vi "Prompt for Step.vi"(8 "error in (no error)":errorcluster, 10 "Subpanel Ref":refnum<vi>, 11 "Numeric Assertion in":refnum<class "Numeric Assertion.lvclass">) -> (0 "error out":errorcluster, 3 "Numeric Assertion out":refnum<class "Numeric Assertion.lvclass">)   [LabVIEW 2020, in "MacroAssert.lvlib" / "Numeric Assertion.lvclass"]
doc: "Displays its own window into <B>Subpanel Ref</B> for the user to enter a macro step."
uses:
  Numeric Assertion.lvclass
  Assertion Step/Assertion Step.lvclass
panel:
  out "Subtype Description":string
  in  "Comparison Value":dbl
  in  "Comparison Type":u16(ring) items=["Equals", "Is greater than", "Is greater than or equal to", "Is less than", "Is less than or equal to", "Does not equal"]
  in  "Step Subtype":u16(ring) items=["Numeric Ctl Value", "Array Ctl Size", "Ctl Width Property", "Ctl Height Property", "VI Width", "VI Height", "Window Width", "Window Height", "Window Scale"]
  in  "Object Name":string
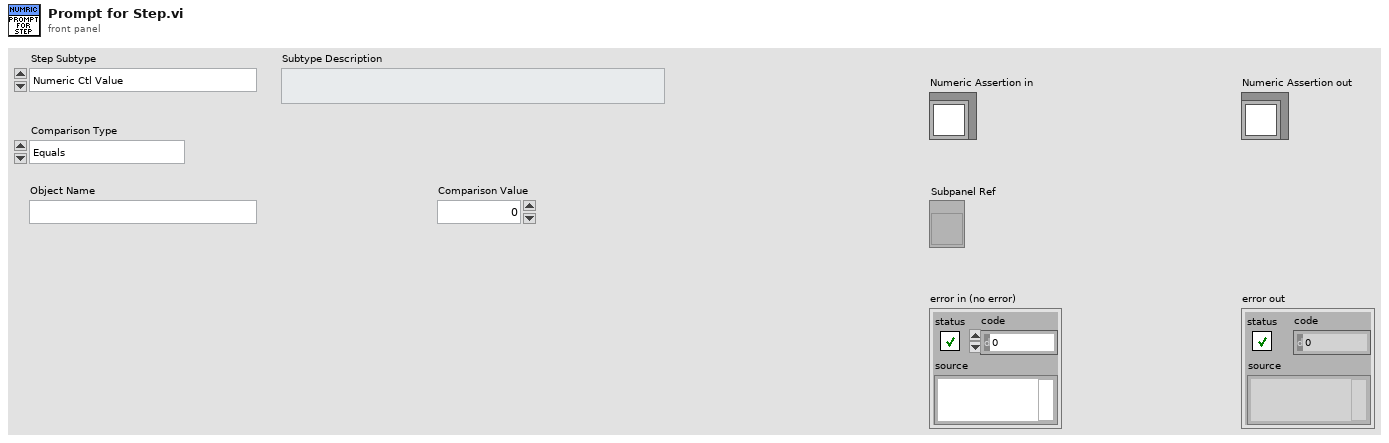
[diagram p1: front panel]
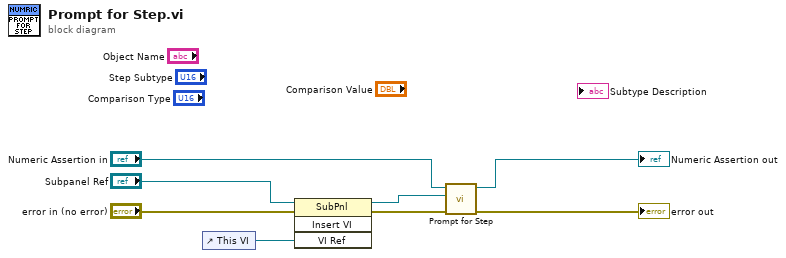
[diagram p0: block diagram]
diagram:
  n1 = control-ref of="This VI"() -> (w6:refnum<vi>)
  n2 = invoke class="SubPnl" method="Insert VI"(reference="Subpanel Ref", error in="error in (no error)", "VI Ref"=w6) -> (reference out=w7:refnum<vi>, error out=w8:errorcluster)  [unwired: 1 in, 2 out]
  n3 = call-parent "Prompt for Step.vi"("error in (no error)"=w8, "Subpanel Ref"=w7, "Step in"="Numeric Assertion in") -> ("error out"=→"error out":errorcluster, "Step out"=→"Numeric Assertion out":refnum<class "Numeric Assertion.lvclass">)  [unwired: 7 in]
